vi "Judge.vi"(6 "mediaplayer":refnum<k7>, 7 "error in (no error)":errorcluster, 8 "Road Refnum":refnum<vi>, 9 "Coin Refnum":refnum<vi>, 10 "Player Refnum":refnum<vi>) -> (0 "error out":errorcluster, 1 "Score":u16, 2 "roadnext":i32, 3 "coinnext":i32, 4 "Action":enum16{"Cat", "Jump", "Fall", "Fly", "Rote"}(ring))   [LabVIEW 2010]
panel:
  in  "Coin":u16(ring)
  in  "Player":u16(ring)
  in  "road":u16(ring)
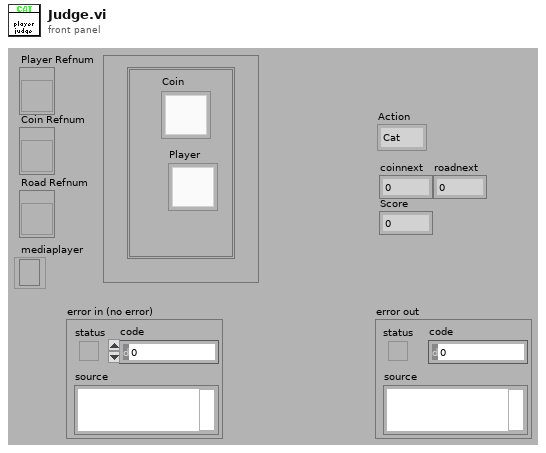
[diagram p1: front panel]
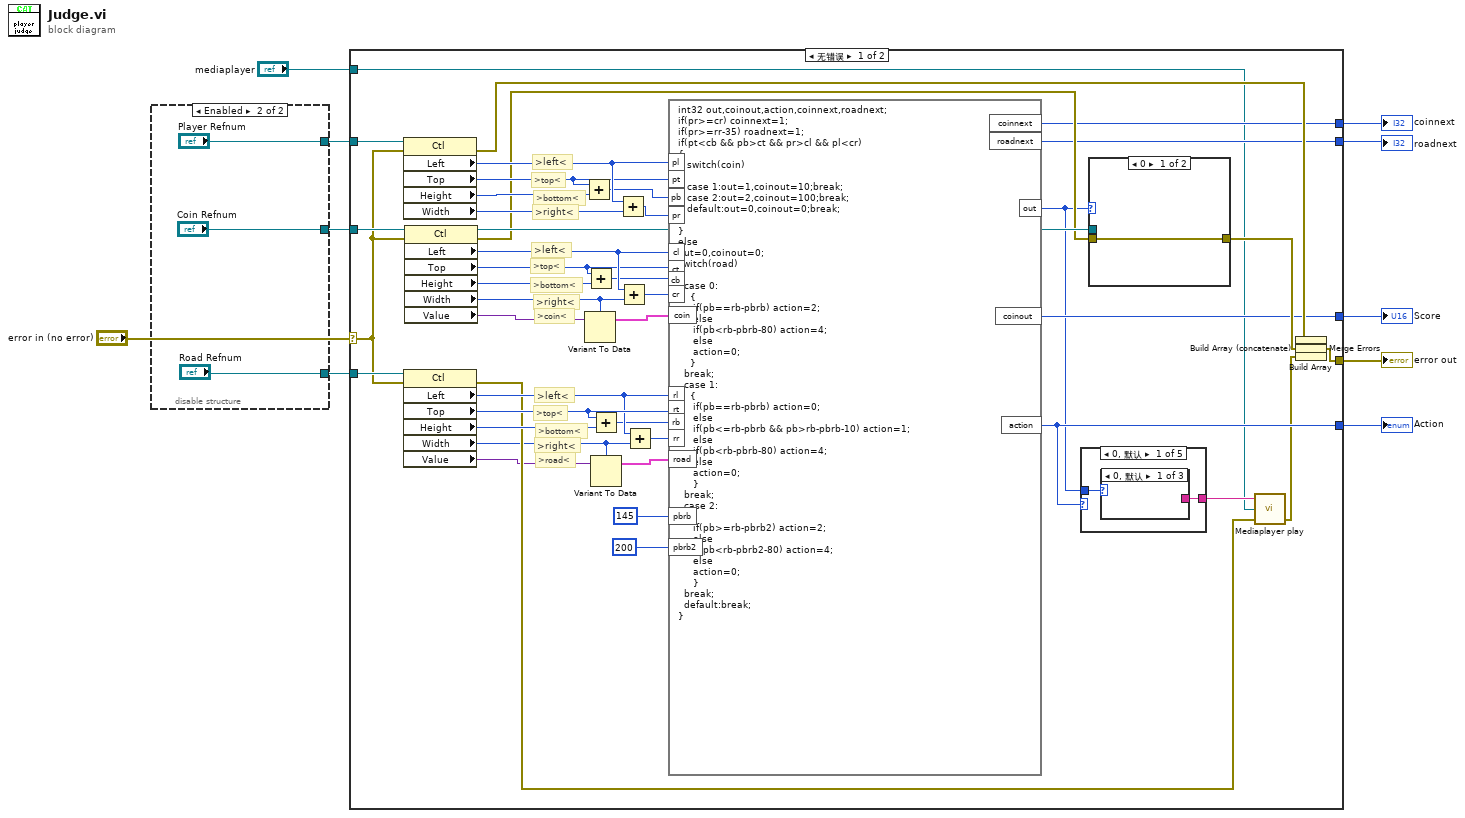
[diagram p0: block diagram]
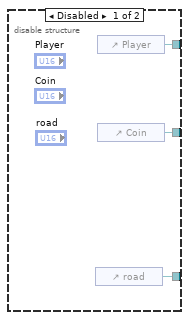
[diagram p2: hidden frame]
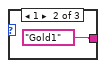
[diagram p3: hidden frame]
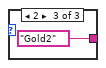
[diagram p4: hidden frame]
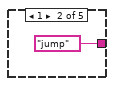
[diagram p5: hidden frame]
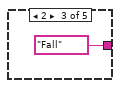
[diagram p6: hidden frame]
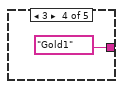
[diagram p7: hidden frame]
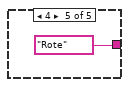
[diagram p8: hidden frame]
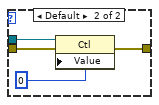
[diagram p9: hidden frame]
diagram:
  n1 = disable-structure shown="Enabled" {
    disable-tunnel: [w13 "Player Refnum"] -> w10
    disable-tunnel: [w12 "Coin Refnum"] -> w9
    disable-tunnel: [w11 "Road Refnum"] -> w8
    frame Disabled {
      n2 = control-ref of="road"() -> (w11:refnum<vi>)
      n3 = control-ref of="Player"() -> (w13:refnum<vi>)
      n4 = control-ref of="Coin"() -> (w12:refnum<vi>)
    }
    frame Enabled {
    }
  }
  n5 = case shown="无错误" "error in (no error)" {
    selector: "error in (no error)" -> [w44 w74]
    tunnel: w10 -> [w60 _]
    tunnel: w9 -> [w59 _]
    tunnel: w8 -> [w47 _]
    tunnel: [w41 w74] -> w6
    tunnel: [w26 _] -> w2
    tunnel: [w33 _] -> w5
    tunnel: [w32 _] -> w4
    tunnel: [w31 _] -> w3
    tunnel: "mediaplayer" -> [w23 _]
    frame No Error {
      # ">road<"
      # ">right<"
      # ">bottom<"
      # ">top<"
      # ">left<"
      # ">coin<"
      # ">right<"
      # ">bottom<"
      # ">top<"
      # ">right<"
      # ">bottom<"
      # ">top<"
      # ">left<"
      # ">left<"
      n6 = property class="Ctl"(reference=w60, error in=w44) -> (error out=w43:errorcluster, "Left"=w55:i32, "Top"=w54:i32, "Height"=w58:u32, "Width"=w57:u32)  [unwired: 1 out]
      n7 = property class="Ctl"(reference=w47, error in=w44) -> (error out=w22:errorcluster, "Left"=w37:i32, "Top"=w38:i32, "Height"=w39:u32, "Width"=w18:u32, "Value"=w19:variant)  [unwired: 1 out]
      n8 = property class="Ctl"(reference=w59, error in=w44) -> (reference out=w46:refnum<vi>, error out=w45:errorcluster, "Left"=w51:i32, "Top"=w50:i32, "Height"=w56:u32, "Width"=w29:u32, "Value"=w40:variant)
      n9 = Add(x=w54, y=w58) -> (x+y=w53:u32)
      n10 = Variant To Data(Variant=w40, type=w29) -> (data=w30:cluster{})  [unwired: 1 in, 1 out]
      n11 = Add(x=w50, y=w56) -> (x+y=w49:u32)
      n12 = Add(x=w38, y=w39) -> (x+y=w36:u32)
      n13 = Variant To Data(Variant=w19, type=w18) -> (data=w28:cluster{})  [unwired: 1 in, 1 out]
      n14 = Add(x=w55, y=w57) -> (x+y=w52:u32)
      n15 = Add(x=w51, y=w29) -> (x+y=w48:u32)
      n16 = Add(x=w37, y=w18) -> (x+y=w35:u32)
      n17 = formula code="int32 out,coinout,action,coinnext,roadnext;\nif(pr>=cr) coinnext=1; \nif(pr>=rr-35) roadnext=1;\nif(pt<cb && pb>ct && pr>cl && pl<cr)\n{\n   switch(coin)\n{\n   case 1:out=1,coinout=10;break;\n   case 2:out=2,coinout=100;break;\n   default:out=0,coinout=0;break;\n}\n}\nelse\nout=0,coinout=0;\nswitch(road)\n{\n  case 0:\n    {\n     if(pb==rb-pbrb) action=2;\n     else\n     if(pb<rb-pbrb-80) action=4;\n     else\n     action=0;\n    } \n  break;\n  case 1:\n    {\n     if(pb==rb-pbrb) action=0;\n     else\n     if(pb<=rb-pbrb && pb>rb-pbrb-10) action=1;\n     else\n     if(pb<rb-pbrb-80) action=4;\n     else\n     action=0;\n     }\n  break;\n  case 2:\n    {\n     if(pb>=rb-pbrb2) action=2;\n     else\n     if(pb<rb-pbrb2-80) action=4;\n     else\n     action=0;\n     }\n  break;\n  default:break;\n}"("pl"=w55, "pt"=w54, "pb"=w53, "pr"=w52, "cl"=w51, "ct"=w50, "cb"=w49, "cr"=w48, "coin"=w30, "rl"=w37, "rt"=w38, "rb"=w36, "rr"=w35, "road"=w28, "pbrb"=145, "pbrb2"=200) -> ("out"=w25:i32, "coinout"=w31:i32, "action"=w26:i32, "coinnext"=w33:i32, "roadnext"=w32:i32)
      n18 = case shown="0, 默认" w26 {
        tunnel: w25 -> [w62 _ _ _ _]
        tunnel: [w61 "jump" ("music") "Fall" ("music") "Gold1" ("music") "Rote" ("music")] -> w24
        frame 0, Default {
          n19 = case shown="0, 默认" w62 {
            tunnel: [_ "Gold1" ("music") "Gold2" ("music")] -> w61
            frame 0, Default {
            }
            frame 1 {
            }
            frame 2 {
            }
          }
        }
        frame 1 {
        }
        frame 2 {
        }
        frame 3 {
        }
        frame 4 {
        }
      }
      n20 = case shown="0" w25 {
        tunnel: w46 -> [_ w73]
        tunnel: w45 -> [w69 w72]
        tunnel: [w69 w71] -> w42
        frame 0 {
        }
        frame Default {
          n21 = property class="Ctl"(reference=w73, error in=w72, "Value"=u16 0) -> (error out=w71:errorcluster)  [unwired: 1 out]
        }
      }
      n22 = call "Mediaplayer play.vi"("music"=w24, "MediaPlayer"=w23, "error in"=w22) -> ("error out"=w21:errorcluster)  [unwired: 4 in]
      n23 = Build Array(w43, w42, w21) -> (w34:errorcluster[])
      n24 = Build Array (concatenate)(w34) -> (w27:errorcluster[])
      n25 = Merge Errors(w27) -> (w41:errorcluster)
    }
    frame Error {
    }
  }
  "Score" <- w3
  "error out" <- w6
  "coinnext" <- w5
  "roadnext" <- w4
  "Action" <- w2
